vi "ResponseActionTemplate.vi"(7 "HTTP_address":string, 8 "error in (no error)":errorcluster, 10 "Value":T2, 11 "Refnum in":T1) -> (0 "error out":errorcluster)   [LabVIEW 2016]
uses:
  cgi_string.ctl
  <vilib>/httpClient/ClientHandle.ctl
  <vilib>/httpClient/LabVIEWHTTPClient.lvlib
types:
  T1 = typedef "LabVIEWHTTPClient.lvlib/ClientHandle.ctl" = refnum<k1>
  T2 = typedef "cgi_string.ctl" = string
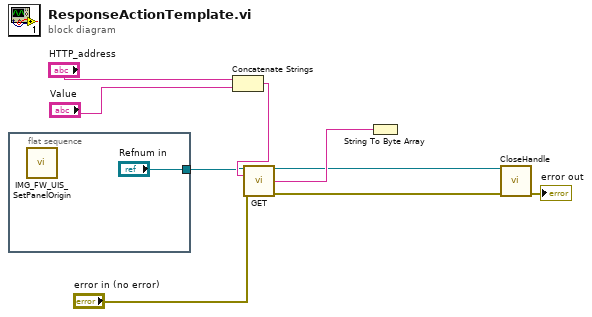
[diagram p0: block diagram]
diagram:
  n1 = flat-sequence {
    tunnel: ["Refnum in"] -> w6
    frame #0 {
      n2 = call "IMG_FW_UIS_SetPanelOrigin.vi"() -> ()  [unwired: 11 in, 1 out]
    }
  }
  n3 = Concatenate Strings("HTTP_address", "Value") -> (w9:string)
  n4 = call <vilib>:"GET.vi"("client handle"=w6, "url"=w9, "error in (no error)"="error in (no error)") -> ("client handle out"=w3:T1, "body"=w5:string, "error out"=w4:errorcluster)  [unwired: 9 in, 1 out]
  n5 = String To Byte Array(string=w5) -> ()  [unwired: 1 out]
  n6 = call <vilib>:"CloseHandle.vi"("client handle"=w3, "error in (no error)"=w4) -> ("error out"=→"error out":errorcluster)  [unwired: 13 in]
